vi "IEEE_11073.vi"(10 "Message":u8[](array[numeric])) -> (0 "10^x":dbl, 2 "Body Temperature, deg C":dbl, 8 "Power":i8)   [LabVIEW 2015]
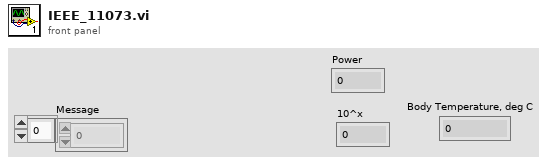
[diagram p1: front panel]
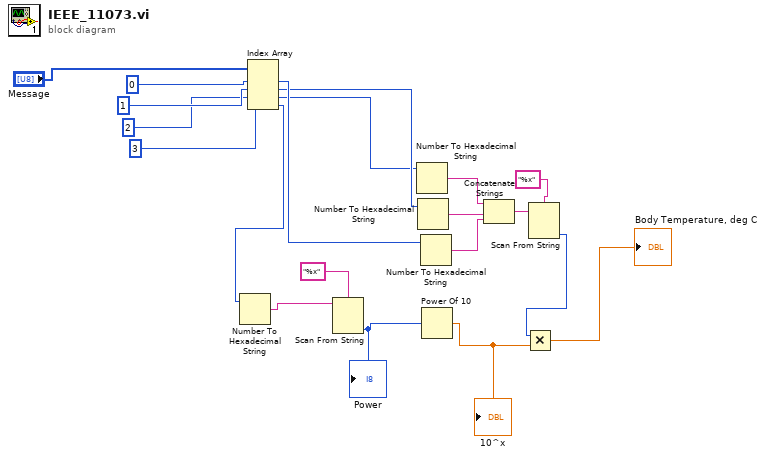
[diagram p0: block diagram]
diagram:
  n1 = Index Array(array="Message", index #1=0 ("index"), index #2=1 ("index"), index #3=2 ("index"), index #4=3 ("index")) -> (element #1=w3:u8, element #2=w2:u8, element #3=w1:u8, element #4=w4:u8)
  n2 = Number To Hexadecimal String(2:w4) -> (0:w18:string)  [unwired: 1 in]
  n3 = Scan From String(format string="%x", input string=w18) -> (output 1=w19:i8)  [unwired: 3 in, 3 out]
  "Power" <- w19
  n4 = Number To Hexadecimal String(2:w1) -> (0:w16:string)  [unwired: 1 in]
  n5 = Number To Hexadecimal String(2:w2) -> (0:w15:string)  [unwired: 1 in]
  n6 = Number To Hexadecimal String(2:w3) -> (0:w14:string)  [unwired: 1 in]
  n7 = Power Of 10(x=w19) -> (10^x=w17:dbl)
  "10^x" <- w17
  n8 = Concatenate Strings(w16, w15, w14) -> (w10:string)
  n9 = Scan From String(format string="%x", input string=w10) -> (output 1=w12:u32)  [unwired: 3 in, 3 out]
  n10 = Multiply(x=w12, y=w17) -> (x*y=→"Body Temperature, deg C":dbl)
